vi "UpdateServerAddress.vi"(8 "error in (no error)":errorcluster, 10 "Server address":string, 11 "TCP_serverGUI in":refnum<class "TCP_serverGUI.lvclass">) -> (0 "error out":errorcluster, 3 "TCP_serverGUI out":refnum<class "TCP_serverGUI.lvclass">)   [LabVIEW 2023, in "TCP_serverGUI.lvlib" / "TCP_serverGUI.lvclass"]
uses:
  TCP_serverGUI.lvclass
  TCP_serverGUI.lvclass/TCP_serverGUI.ctl
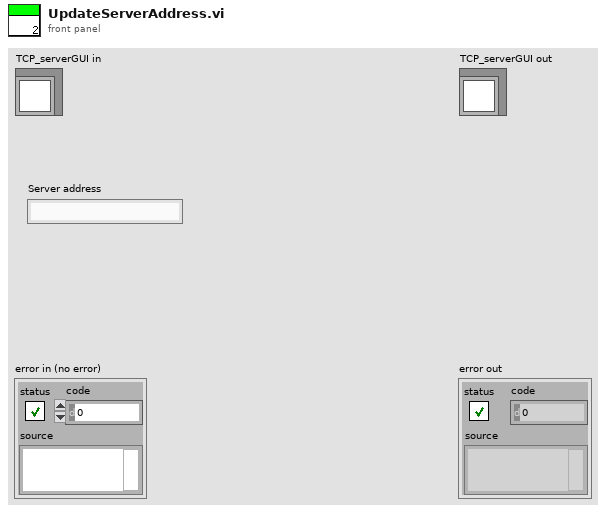
[diagram p1: front panel]
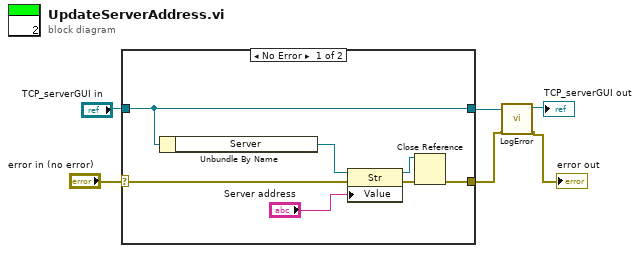
[diagram p0: block diagram]
diagram:
  n1 = case shown="No Error" "error in (no error)" {
    selector: "error in (no error)" -> [w10 w15]
    tunnel: [w7 w15] -> w2
    tunnel: [w13 w14] -> w4
    tunnel: "TCP_serverGUI in" -> [w13 w14]
    frame No Error {
      n2 = Unbundle By Name(w13) -> ("Server"=w12:refnum<vi>)
      n3 = property class="Str"(reference=w12, error in=w10, "Value"="Server address") -> (reference out=w8:refnum<vi>, error out=w9:errorcluster)
      n4 = Close Reference(reference=w8, error in (no error)=w9) -> (error out=w7:errorcluster)
    }
    frame Error {
    }
  }
  n5 = call "LogError.vi"("error in (no error)"=w2, "TCP_serverGUI in"=w4) -> ("error out"=→"error out":errorcluster, "TCP_serverGUI out"=→"TCP_serverGUI out":refnum<class "TCP_serverGUI.lvclass">)  [unwired: 8 in]
